vi "Tosca-Write Parameters.vi"(0 "Path in":path, 5 "Tosca":refnum<class "Parameters.lvclass">, 7 "FSM.Graph":refnum<class "FSM.Graph.lvclass">, 11 "error in (no error)":errorcluster, 12 "Prompt (T)":bool=TRUE) -> (4 "Path out":path, 8 "Saved?":bool, 15 "error out":errorcluster)   [LabVIEW 2020]
uses:
  Classes/Parameters/Parameters.lvclass
  FSM Graph VIs/LV Source/Classes/FSM.Graph/FSM.Graph.lvclass
  Sub VIs/Tosca-Globals.vi
panel:
  in  "Metadata":cluster{"Version":string}
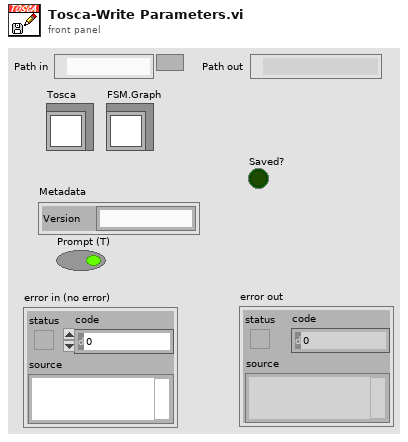
[diagram p1: front panel]
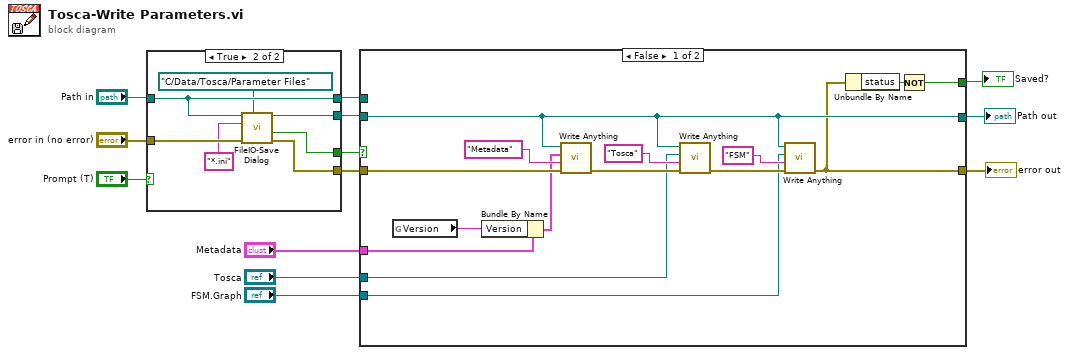
[diagram p0: block diagram]
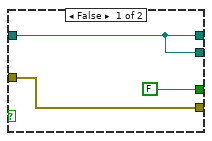
[diagram p2: hidden frame]
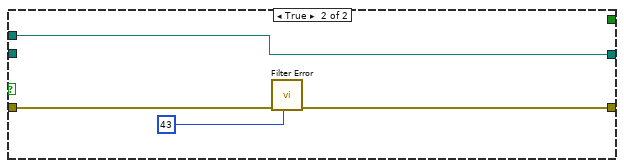
[diagram p3: hidden frame]
diagram:
  n1 = case shown="True" "Prompt (T)" {
    tunnel: "error in (no error)" -> [w14 w23]
    tunnel: [FALSE ("cancelled") w22] -> w12
    tunnel: [w16 w21] -> w11
    tunnel: [w14 w20] -> w9
    tunnel: "Path in" -> [w16 w18]
    tunnel: [w16 w18] -> w5
    frame False {
    }
    frame True {
      n2 = call "FileIO-Save Dialog.vi"("Default Folder"=path "C:/Data/Tosca/Parameter Files", "error in"=w23, "pattern (all files)"="*.ini", "Start path"=w18) -> ("error out"=w20:errorcluster, "cancelled"=w22:bool, "selected path"=w21:path)  [unwired: 5 in]
    }
  }
  n3 = case shown="False" w12 {
    tunnel: [w31 w41] -> w10
    tunnel: w11 -> [w31 _]
    tunnel: w9 -> [w37 w42]
    tunnel: w5 -> [_ w41]
    tunnel: [w29 w40] -> w7
    tunnel: "Tosca" -> [w24 _]
    tunnel: [w27 _] -> w4
    tunnel: "Metadata" -> [w34 _]
    tunnel: "FSM.Graph" -> [w26 _]
    frame False {
      n4 = global read "Tosca-Globals.vi" "Version"() -> (w25:string)
      n5 = Bundle By Name(cluster=w34, "Version"=w25) -> (w33:cluster{"Version":string})
      n6 = call "Write Anything.vi"("Error In"=w37, "Section Name (Name of \"Anything\")"="Metadata", "Anything"=w33, "Path (dialog)"=w31) -> ("Error Out"=w36:errorcluster)  [unwired: 6 in, 1 out]
      n7 = call "Write Anything.vi"("Error In"=w36, "Section Name (Name of \"Anything\")"="Tosca" ("Section Name (Name of \"Anything\")"), "Anything"=w24, "Path (dialog)"=w31) -> ("Error Out"=w32:errorcluster)  [unwired: 6 in, 1 out]
      n8 = call "Write Anything.vi"("Error In"=w32, "Section Name (Name of \"Anything\")"="FSM" ("Section Name (Name of \"Anything\")"), "Anything"=w26, "Path (dialog)"=w31) -> ("Error Out"=w29:errorcluster)  [unwired: 6 in, 1 out]
      n9 = Unbundle By Name(w29) -> ("status"=w28:bool)
      n10 = Not(x=w28) -> (.not. x?=w27:bool)
    }
    frame True {
      n11 = call "Filter Error.vi"("error in (no error)"=w42, "code to ignore"=43) -> ("error out"=w40:errorcluster)  [unwired: 9 in]
    }
  }
  "error out" <- w7
  "Path out" <- w10
  "Saved?" <- w4
